vi "MGCC_Resync_global.vi"() -> ()   [LabVIEW 2016]
panel:
  in  "b_MGCC_Resync_Enable":bool[](array[boolean])
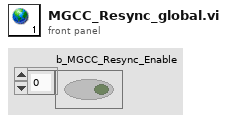
[diagram p1: front panel]
diagram:
